vi "ConfigDialog.vi"(4 "Severity (Critical)":string="Critical", 6 "Priority (2)":u8=2, 7 "reference":refnum<vi>, 8 "ErrorIn Array":errorcluster[](array[cluster]), 11 "Instrument Modules New In":T1=[{"PluginSelection"=4, "ConfigDialog"=FALSE}]) -> (0 "ErrorOut Array":errorcluster[](array[cluster]), 3 "Instrument Modules Out":T1=[{"PluginSelection"=4, "ConfigDialog"=FALSE}])   [LabVIEW 2018]
doc: "This VI opens the Preference Dialog for the selected module."
uses:
  Framework/InstrumentModulesControl.ctl
  NistPluggableModules/BusClass/Bus.lvclass/Bus.ctl
  NistPluggableModules/BusClass/Accessors/Read Test.vi
  NistPluggableModules/TestClass/Test.lvclass
  NistPluggableModules/BusClass/Bus.lvclass
  <userlib>/NIST/NISTErrorLib/NISTErrorLib.lvlib
  Queue/Queue.lvlib
panel:
  in  "Instrument Modules Old In":T1=[{"PluginSelection"=4, "ConfigDialog"=FALSE}]
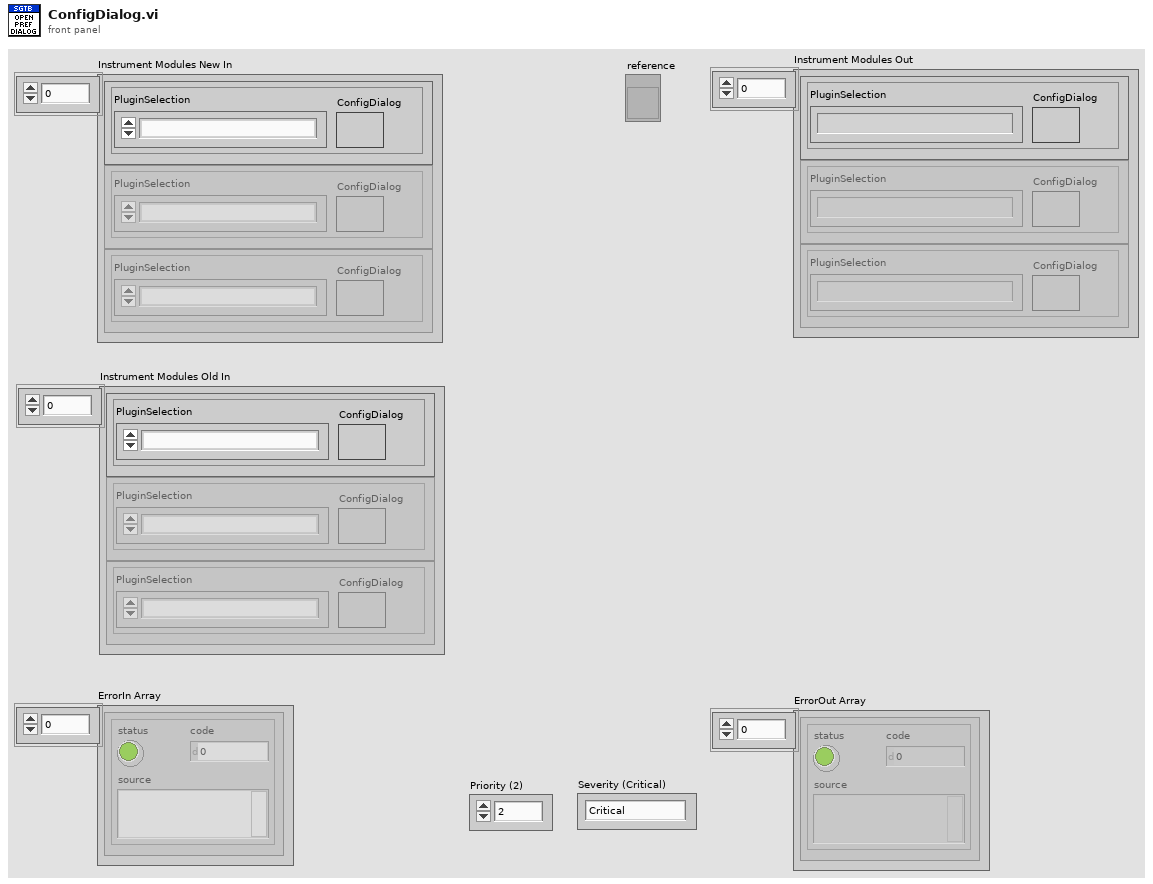
[diagram p1: front panel]
types:
  T1 = typedef "InstrumentModulesControl.ctl" = cluster{"PluginSelection":u16, "ConfigDialog":bool}[]
  T2 = cluster{"PluginSelection":u16, "ConfigDialog":bool}
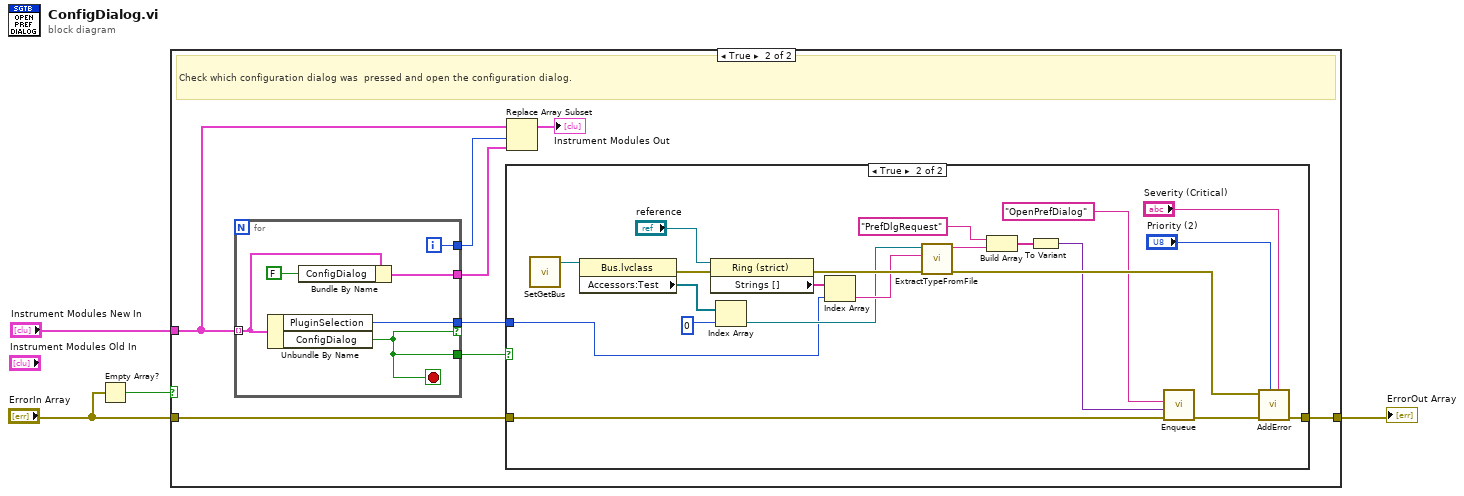
[diagram p0: block diagram]
diagram:
  n1 = Empty Array?(array="ErrorIn Array") -> (empty?=w1:bool)
  n2 = case shown="True" w1 {
    tunnel: [w5 w13] -> w4
    tunnel: "Instrument Modules New In" -> [_ w9]
    tunnel: "ErrorIn Array" -> [w5 w12]
    frame False {
      # "If error was passed in take no action."
    }
    frame True {
      # "Check which configuration dialog was  pressed and open the configuration dialog."
      n3 = for {
        tunnel: w9 -> [w19] mode=indexing
        tunnel: [w17] -> w7
        tunnel: [w16] -> w11 if=w15
        tunnel: [w15] -> w10
        tunnel: [w14] -> w8
        i -> [w14]
        stop <- w15 stop-if-true
        n4 = Unbundle By Name(w19) -> ("PluginSelection"=w16:u16, "ConfigDialog"=w15:bool)
        n5 = Bundle By Name(cluster=w19, "ConfigDialog"=FALSE ("ConfigDialog 2")) -> (w17:T2)
      }
      n6 = case shown="True" w10 {
        tunnel: [w20 w41] -> w13
        tunnel: w12 -> [w20 w32]
        tunnel: w11 -> [_ w29]
        frame False {
        }
        frame True {
          n7 = call "SetGetBus.vi"() -> ("Bus.lvclass"=w40:refnum<class "Bus.lvclass">)  [unwired: 11 in]
          n8 = property class="Bus.lvclass"(reference=w40) -> (error out=w35:errorcluster, "Accessors:Test"=w33:refnum<class "Test.lvclass">[])  [unwired: 1 in, 1 out]
          n9 = property class="Ring (strict)"(reference="reference", error in=w35) -> (error out=w37:errorcluster, "Strings []"=w38:string[])  [unwired: 1 out]
          n10 = Index Array(array=w33, index=0) -> (element=w30:refnum<class "Test.lvclass">)
          n11 = Index Array(array=w38, index=w29) -> (element=w36:string)
          n12 = call "ExtractTypeFromFile.vi"("error in (no error)"=w37, "Type"=w36, "Test in"=w30) -> ("error out"=w25:errorcluster, "PluginType"=w31:string)  [unwired: 7 in]
          n13 = Build Array("PrefDlgRequest" ("string"), w31) -> (w22:string[])
          n14 = To Variant(anything=w22) -> (Variant=w21:variant)
          n15 = call "Enqueue.vi"("ErrorArray"=w32, "Message Data"=w21, "Message"="OpenPrefDialog") -> ("ErrorArray"=w26:errorcluster[])  [unwired: 8 in]
          n16 = call <userlib>:"AddError.vi"("Severity"="Severity (Critical)", "Priority"="Priority (2)", "ErrorArray"=w26, "error in (no error)"=w25) -> ("ErrorArray"=w41:errorcluster[])  [unwired: 6 in, 1 out]
        }
      }
      n17 = Replace Array Subset(array=w9, new element=w7, index=w8) -> (→"Instrument Modules Out":T1)
    }
  }
  "ErrorOut Array" <- w4
